vi "youtube search.vi"() -> ()   [LabVIEW 2020]
panel:
  in  "Youtube Search Query":string
  in  "SHDocVw.IWebBrowser2":refnum<k7>
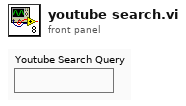
[diagram p1: front panel]
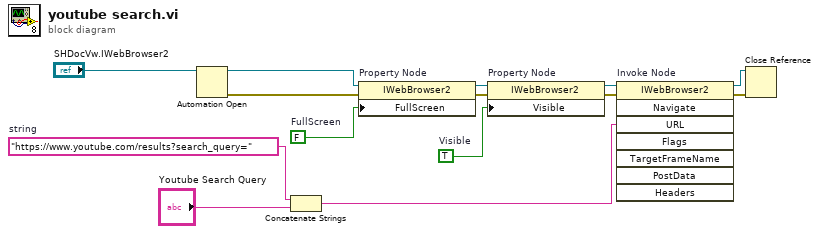
[diagram p0: block diagram]
diagram:
  w4 = "https://www.youtube.com/results?search_query="  # string
  w8 = TRUE  # Visible
  w9 = FALSE  # FullScreen
  n1 = Automation Open(Automation Refnum="SHDocVw.IWebBrowser2") -> (Automation Refnum=w13:refnum<k7>, error out=w12:errorcluster)  [unwired: 3 in]
  n2 = Concatenate Strings "Concatenate Strings"(w4, "Youtube Search Query") -> (w5:string)
  n3 = property on="Property Node" class="IWebBrowser2"(reference=w13, error in=w12, "FullScreen"=w9) -> (reference out=w11:refnum<k7>, error out=w10:errorcluster)
  n4 = property on="Property Node" class="IWebBrowser2"(reference=w11, error in=w10, "Visible"=w8) -> (reference out=w7:refnum<k7>, error out=w6:errorcluster)
  n5 = invoke on="Invoke Node" class="IWebBrowser2" method="Navigate"(reference=w7, error in=w6, "URL"=w5) -> (reference out=w2:refnum<k7>, error out=w1:errorcluster)  [unwired: 5 in, 6 out]
  n6 = Close Reference(reference=w2, error in (no error)=w1) -> ()  [unwired: 1 out]
